vi "UI_Test_Template_Modify.vi"() -> ()   [LabVIEW 2014]
panel:
  out "载荷谱列表":string[][](table)
  in  "退出":bool
  in  "选项卡控件":enum32{"添加模板", "删除模板", "修改模板"}(tab)
  in  "添加模板":bool
  in  "请输入模板名称":string
  in  "添加载荷谱模板":string[][](table)
  in  "删除模板":bool
  in  "请输入要删除的模板名称":string
  out "模板详情":string[][](table)
  in  "删除模板查询":bool
  in  "保存修改":bool
  in  "修改模板查询":bool
  in  "请输入修改的的模板名称":string
  in  "修改载荷谱模板":string[][](table)
  # "载荷谱模板维护"
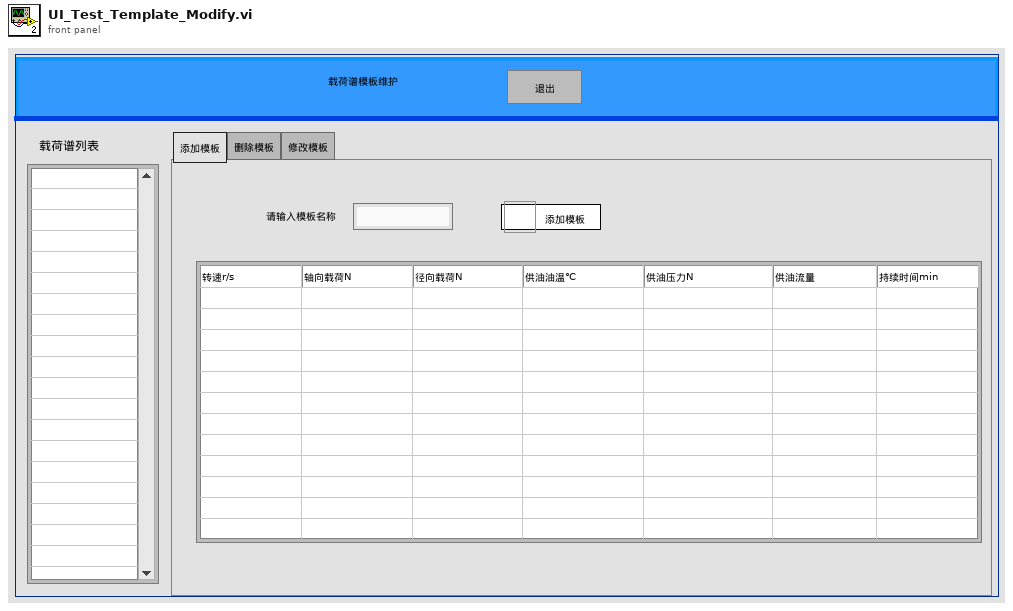
[diagram p1: front panel]
types:
  T1 = typedef "LVPoint32TypeDef.ctl" = cluster{"Horizontal":i32, "Vertical":i32}
  T2 = typedef "LVRowAndColumnTypeDef.ctl" = cluster{"Row":i32, "Column":i32}
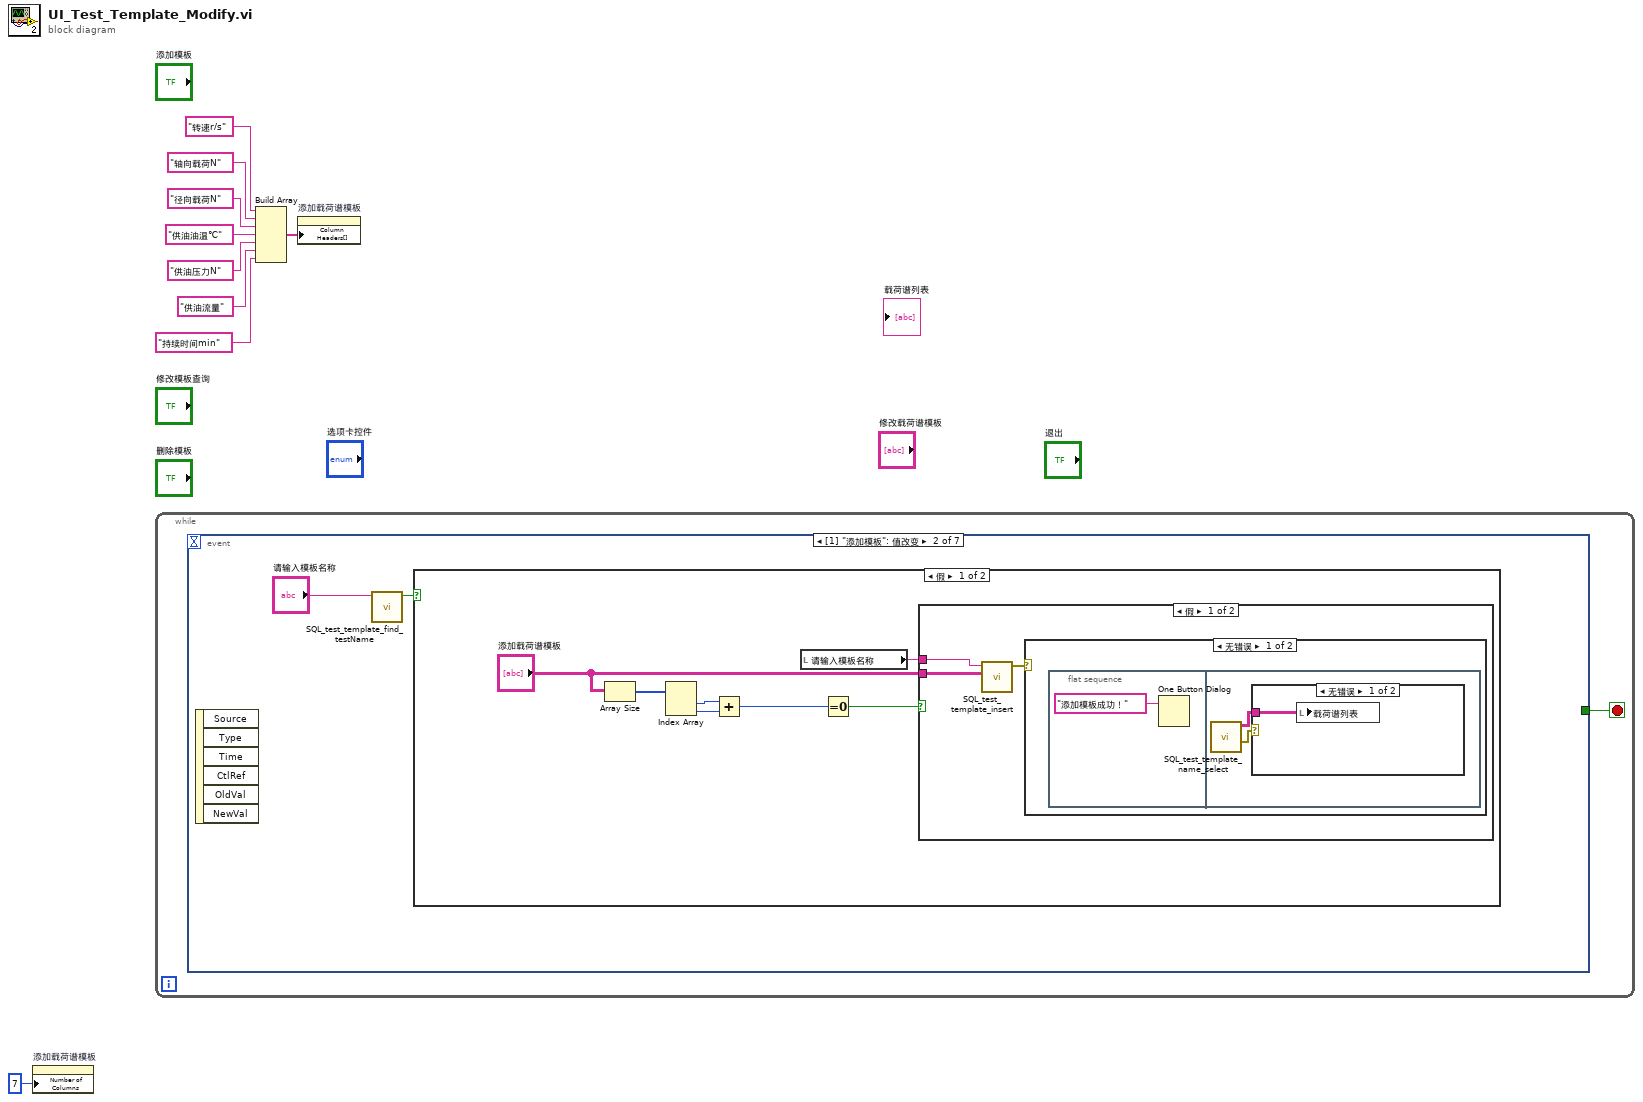
[diagram p0: block diagram]
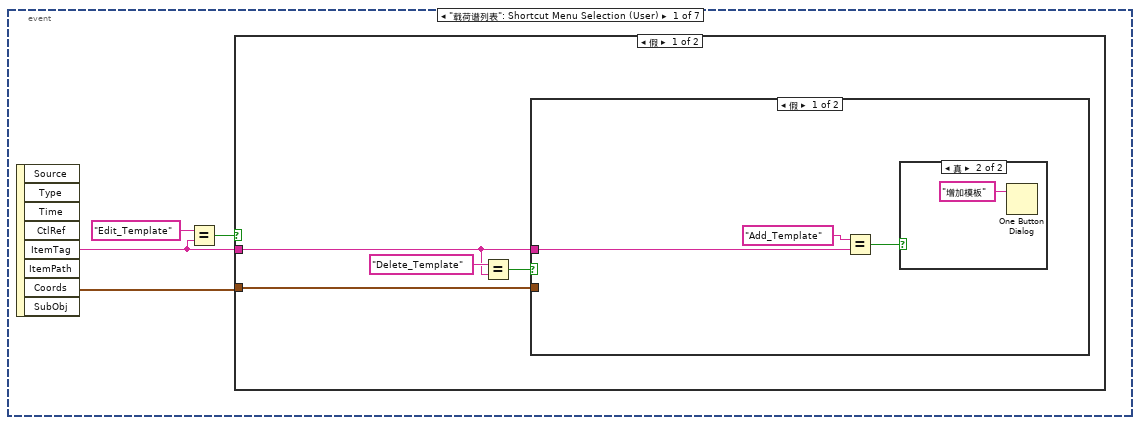
[diagram p2: hidden frame]
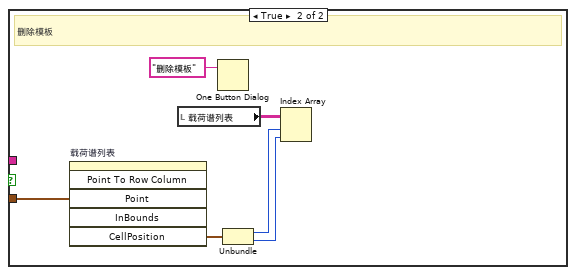
[diagram p4: hidden frame]
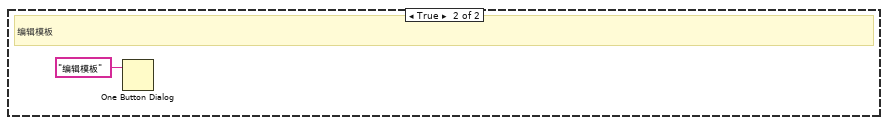
[diagram p5: hidden frame]
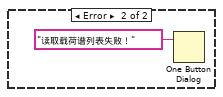
[diagram p6: hidden frame]
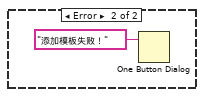
[diagram p7: hidden frame]
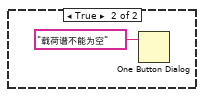
[diagram p8: hidden frame]
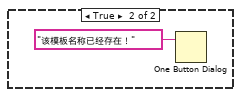
[diagram p9: hidden frame]
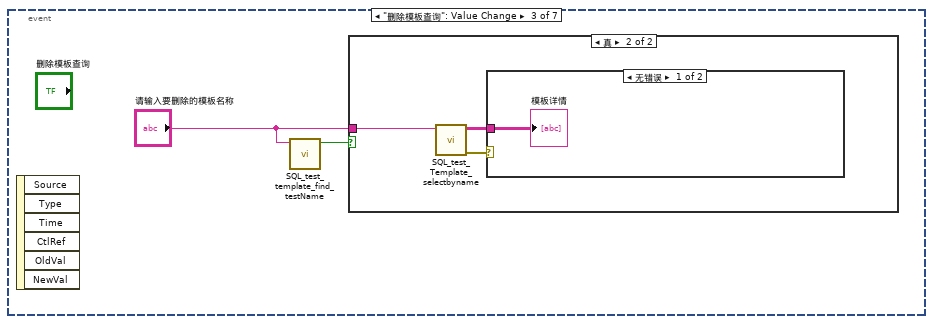
[diagram p10: hidden frame]
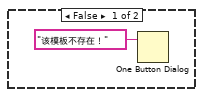
[diagram p11: hidden frame]
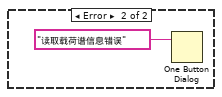
[diagram p12: hidden frame]
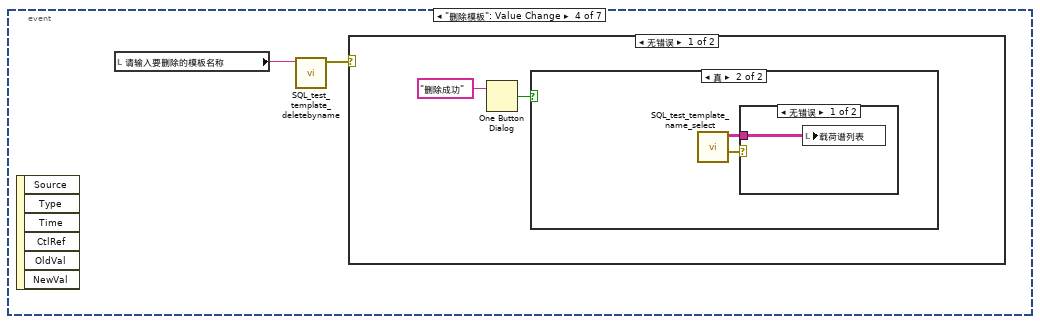
[diagram p13: hidden frame]
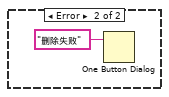
[diagram p16: hidden frame]
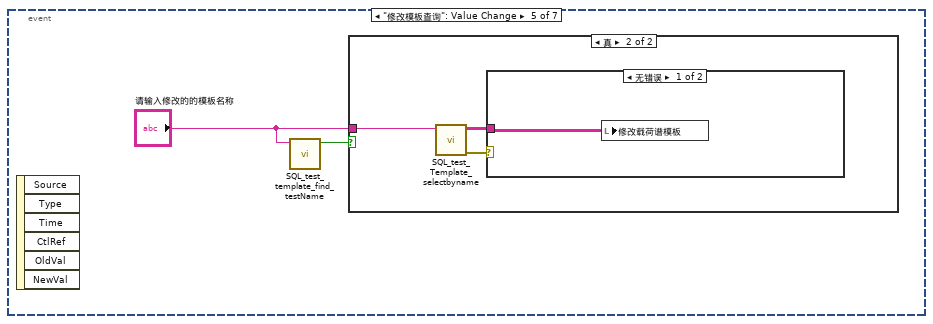
[diagram p17: hidden frame]
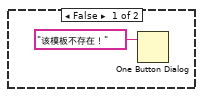
[diagram p18: hidden frame]
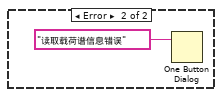
[diagram p19: hidden frame]
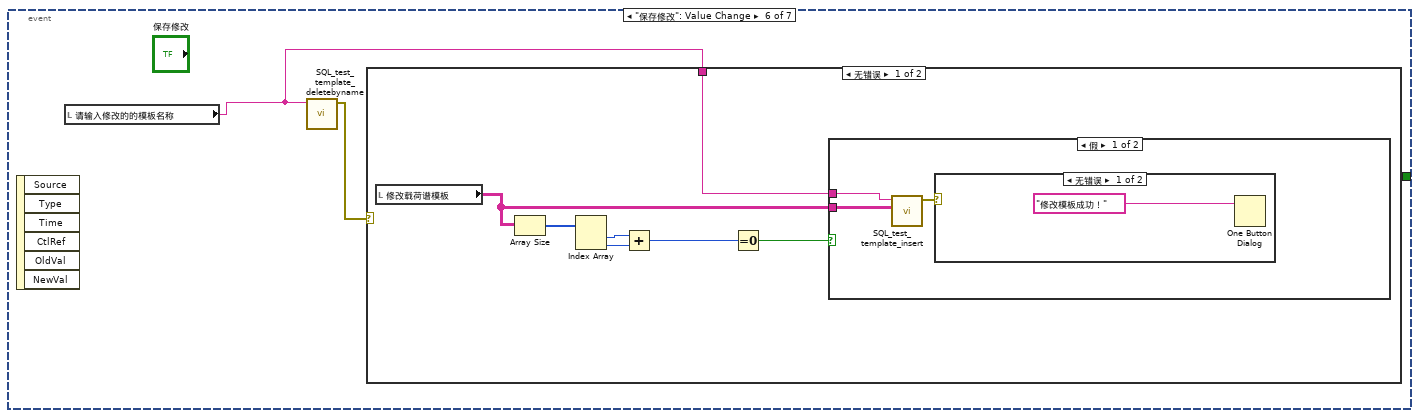
[diagram p20: hidden frame]
diagram:
  n1 = property on="添加载荷谱模板" class="Tbl (严格)"("Number of Columns"=u32 7 ("列数")) -> ()  [unwired: 2 in, 2 out]
  n2 = while {
    stop <- w10 stop-if-true
    n3 = event shown="[1] \"添加模板\": 值改变" {
      selector: _ -> [_ _ _ _ _ _ _]
      dyn-events: _ -> [_ _ _ _ _ _ _]
      timeout: _ -> [_ _ _ _ _ _ _]
      tunnel: [_ _ _ _ _ _ TRUE] -> w10
      event "载荷谱列表": Shortcut Menu Selection (User) {
        n4 = event-data() -> ("ItemTag"=w12:string, "Coords"=w11:T1)  [unwired: 1 in, 6 out]
        n5 = Equal?(x="Edit_Template", y=w12) -> (x = y?=w13:bool)
        n6 = case shown="假" w13 {
          tunnel: w12 -> [w15 _]
          tunnel: w11 -> [w16 _]
          frame False {
            n7 = Equal?(x="Delete_Template", y=w15) -> (x = y?=w17:bool)
            n8 = case shown="假" w17 {
              tunnel: w16 -> [_ w27]
              tunnel: w15 -> [w20 _]
              frame False {
                n9 = Equal?(x="Add_Template", y=w20) -> (x = y?=w19:bool)
                n10 = case shown="真" w19 {
                  frame False {
                  }
                  frame True {
                    n11 = One Button Dialog(message="增加模板" ("消息")) -> ()  [unwired: 1 in, 1 out]
                  }
                }
              }
              frame True {
                # "删除模板"
                n12 = invoke on="载荷谱列表" class="Tbl (严格)" method="Point To Row Column"("Point"=w27) -> ("CellPosition"=w26:T2)  [unwired: 5 in, 5 out]
                n13 = local read "载荷谱列表"() -> (w25:string[][])
                n14 = One Button Dialog(message="删除模板" ("消息")) -> ()  [unwired: 1 in, 1 out]
                n15 = Unbundle(w26) -> ("Row"=w24:i32, "Column"=w23:i32)
                n16 = Index Array(array=w25, index (row)=w24, index (col)=w23) -> ()  [unwired: 1 out]
              }
            }
          }
          frame True {
            # "编辑模板"
            n17 = One Button Dialog(message="编辑模板" ("消息")) -> ()  [unwired: 1 in, 1 out]
          }
        }
      }
      event "添加模板": Value Change {
        n18 = event-data() -> ()  [unwired: 1 in, 6 out]
        n19 = call "SQL_test_template_find_testName.vi"("模板名称"="请输入模板名称") -> ("模板是否存在"=w30:bool)  [unwired: 10 in]
        n20 = case shown="假" w30 {
          frame False {
            n21 = Array Size(array="添加载荷谱模板") -> (size(s)=w38:i32[])
            n22 = Index Array(array=w38) -> (element #1=w37:i32, element #2=w36:i32)  [unwired: 2 in]
            n23 = Add(x=w37, y=w36) -> (x+y=w35:i32)
            n24 = local read "请输入模板名称"() -> (w32:string)
            n25 = Equal To 0?(x=w35) -> (x = 0?=w34:bool)
            n26 = case shown="假" w34 {
              tunnel: "添加载荷谱模板" -> [w40 _]
              tunnel: w32 -> [w39 _]
              frame False {
                n27 = call "SQL_test_template_insert.vi"("表格控件"=w40, "模板名称"=w39) -> ("error out"=w41:errorcluster)  [unwired: 9 in]
                n28 = case shown="无错误" w41 {
                  frame No Error {
                    n29 = flat-sequence {
                      frame #0 {
                        n30 = One Button Dialog(message="添加模板成功！" ("消息")) -> ()  [unwired: 1 in, 1 out]
                      }
                      frame #1 {
                        n31 = call "SQL_test_template_name_select.vi"() -> ("error out"=w44:errorcluster, "模板名称"=w43:string[][])  [unwired: 10 in]
                        n32 = case shown="无错误" w44 {
                          tunnel: w43 -> [w45 _]
                          frame No Error {
                            n33 = local write "载荷谱列表"(w45) -> ()
                          }
                          frame Error {
                            n34 = One Button Dialog(message="读取载荷谱列表失败！" ("消息")) -> ()  [unwired: 1 in, 1 out]
                          }
                        }
                      }
                    }
                  }
                  frame Error {
                    n35 = One Button Dialog(message="添加模板失败！" ("消息")) -> ()  [unwired: 1 in, 1 out]
                  }
                }
              }
              frame True {
                n36 = One Button Dialog(message="载荷谱不能为空" ("消息")) -> ()  [unwired: 1 in, 1 out]
              }
            }
          }
          frame True {
            n37 = One Button Dialog(message="该模板名称已经存在！" ("消息")) -> ()  [unwired: 1 in, 1 out]
          }
        }
      }
      event "删除模板查询": Value Change {
        n38 = event-data() -> ()  [unwired: 1 in, 6 out]
        n39 = call "SQL_test_template_find_testName.vi"("模板名称"="请输入要删除的模板名称") -> ("模板是否存在"=w51:bool)  [unwired: 10 in]
        n40 = case shown="真" w51 {
          tunnel: "请输入要删除的模板名称" -> [_ w53]
          frame False {
            n41 = One Button Dialog(message="该模板不存在！" ("消息")) -> ()  [unwired: 1 in, 1 out]
          }
          frame True {
            n42 = call "SQL_test_Template_selectbyname.vi"("模板名称"=w53) -> ("error out"=w54:errorcluster, "载荷谱信息"=w55:string[][])  [unwired: 9 in]
            n43 = case shown="无错误" w54 {
              tunnel: w55 -> [w56 _]
              frame No Error {
                "模板详情" <- w56
              }
              frame Error {
                n44 = One Button Dialog(message="读取载荷谱信息错误" ("消息")) -> ()  [unwired: 1 in, 1 out]
              }
            }
          }
        }
      }
      event "删除模板": Value Change {
        n45 = event-data() -> ()  [unwired: 1 in, 6 out]
        n46 = local read "请输入要删除的模板名称"() -> (w59:string)
        n47 = call "SQL_test_template_deletebyname.vi"("模板名称"=w59) -> ("error out"=w58:errorcluster)  [unwired: 10 in]
        n48 = case shown="无错误" w58 {
          frame No Error {
            n49 = One Button Dialog(message="删除成功" ("消息")) -> (true=w60:bool)  [unwired: 1 in]
            n50 = case shown="真" w60 {
              frame False {
              }
              frame True {
                n51 = call "SQL_test_template_name_select.vi"() -> ("error out"=w63:errorcluster, "模板名称"=w62:string[][])  [unwired: 10 in]
                n52 = case shown="无错误" w63 {
                  tunnel: w62 -> [w64 _]
                  frame No Error {
                    n53 = local write "载荷谱列表"(w64) -> ()
                  }
                  frame Error {
                  }
                }
              }
            }
          }
          frame Error {
            n54 = One Button Dialog(message="删除失败" ("消息")) -> ()  [unwired: 1 in, 1 out]
          }
        }
      }
      event "修改模板查询": Value Change {
        n55 = event-data() -> ()  [unwired: 1 in, 6 out]
        n56 = call "SQL_test_template_find_testName.vi"("模板名称"="请输入修改的的模板名称") -> ("模板是否存在"=w67:bool)  [unwired: 10 in]
        n57 = case shown="真" w67 {
          tunnel: "请输入修改的的模板名称" -> [_ w69]
          frame False {
            n58 = One Button Dialog(message="该模板不存在！" ("消息")) -> ()  [unwired: 1 in, 1 out]
          }
          frame True {
            n59 = call "SQL_test_Template_selectbyname.vi"("模板名称"=w69) -> ("error out"=w70:errorcluster, "载荷谱信息"=w71:string[][])  [unwired: 9 in]
            n60 = case shown="无错误" w70 {
              tunnel: w71 -> [w72 _]
              frame No Error {
                n61 = local write "修改载荷谱模板"(w72) -> ()
              }
              frame Error {
                n62 = One Button Dialog(message="读取载荷谱信息错误" ("消息")) -> ()  [unwired: 1 in, 1 out]
              }
            }
          }
        }
      }
      event "保存修改": Value Change {
        n63 = event-data() -> ()  [unwired: 1 in, 6 out]
        n64 = local read "请输入修改的的模板名称"() -> (w74:string)
        n65 = call "SQL_test_template_deletebyname.vi"("模板名称"=w74) -> ("error out"=w75:errorcluster)  [unwired: 10 in]
        n66 = case shown="无错误" w75 {
          tunnel: w74 -> [w76 _]
          frame No Error {
            n67 = local read "修改载荷谱模板"() -> (w77:string[][])
            n68 = Array Size(array=w77) -> (size(s)=w82:i32[])
            n69 = Index Array(array=w82) -> (element #1=w81:i32, element #2=w80:i32)  [unwired: 2 in]
            n70 = Add(x=w81, y=w80) -> (x+y=w79:i32)
            n71 = Equal To 0?(x=w79) -> (x = 0?=w78:bool)
            n72 = case shown="假" w78 {
              tunnel: w77 -> [w84 _]
              tunnel: w76 -> [w83 _]
              frame False {
                n73 = call "SQL_test_template_insert.vi"("表格控件"=w84, "模板名称"=w83) -> ("error out"=w85:errorcluster)  [unwired: 9 in]
                n74 = case shown="无错误" w85 {
                  frame No Error {
                    n75 = One Button Dialog(message="修改模板成功！" ("消息")) -> ()  [unwired: 1 in, 1 out]
                  }
                  frame Error {
                    n76 = One Button Dialog(message="修改模板失败！" ("消息")) -> ()  [unwired: 1 in, 1 out]
                  }
                }
              }
              frame True {
                n77 = One Button Dialog(message="载荷谱不能为空" ("消息")) -> ()  [unwired: 1 in, 1 out]
              }
            }
          }
          frame Error {
          }
        }
      }
      event "退出": Value Change {
        n78 = event-data() -> ()  [unwired: 1 in, 6 out]
      }
    }
  }
  n79 = Build Array("转速r/s", "轴向载荷N", "径向载荷N", "供油油温℃", "供油压力N", "供油流量", "持续时间min") -> (w2:string[])
  n80 = property on="添加载荷谱模板" class="Tbl (严格)"("Column Headers[]"=w2) -> ()  [unwired: 2 in, 2 out]
